vi "Send batch otimizado.vi"() -> ()   [LabVIEW 2018]
panel:
  out "delays":u32[](array[numeric])
  out "responses":string[](array[string])
  in  "instructions":string[](array[string])
  out "error out":errorcluster
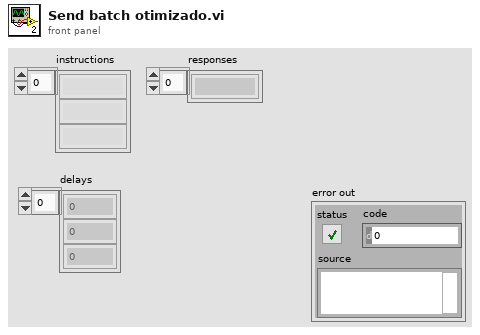
[diagram p1: front panel]
types:
  T1 = enum16{"Standard", "Buffered", "CRLF", "Immediate"}
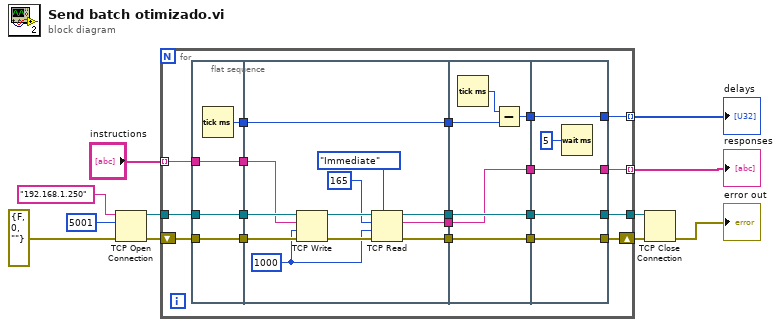
[diagram p0: block diagram]
diagram:
  n1 = TCP Open Connection(address="192.168.1.250" ("motor ip"), remote port or service name=u16 5001 ("motor port"), error in (no error)=errorcluster {"status"=FALSE, "code"=0, "source"=""}) -> (connection ID=w5:refnum<k5>, error out=w9:errorcluster)  [unwired: 2 in]
  n2 = for {
    tunnel: "instructions" -> [w28] mode=indexing
    shift-right: [w12] -> w4
    shift-left: w9 -> [w26]
    tunnel: [w17] -> w10 mode=indexing
    tunnel: w5 -> [w24]
    tunnel: [w20] -> w2
    tunnel: [w19] -> w1 mode=indexing
    n3 = flat-sequence {
      tunnel: [w34] -> w30
      tunnel: w28 -> [w33]
      tunnel: [w33] -> w27
      tunnel: w26 -> [w32]
      tunnel: [w32] -> w25
      tunnel: w24 -> [w31]
      tunnel: [w31] -> w23
      tunnel: [w46] -> w29
      tunnel: w30 -> [w46]
      tunnel: w27 -> [w37]
      tunnel: w25 -> [w42]
      tunnel: w23 -> [w39]
      tunnel: [w41] -> w22
      tunnel: [w38] -> w21
      tunnel: [w35] -> w18
      tunnel: w29 -> [w51]
      tunnel: w22 -> [w49]
      tunnel: w21 -> [w48]
      tunnel: w18 -> [w47]
      tunnel: [w50] -> w16
      tunnel: [w49] -> w15
      tunnel: [w48] -> w14
      tunnel: [w47] -> w13
      tunnel: [w54] -> w19
      tunnel: [w55] -> w20
      tunnel: [w56] -> w12
      tunnel: [w57] -> w17
      tunnel: w16 -> [w57]
      tunnel: w15 -> [w56]
      tunnel: w14 -> [w55]
      tunnel: w13 -> [w54]
      frame #0 {
        n4 = Tick Count (ms)() -> (millisecond timer value=w34:u32)
      }
      frame #1 {
        w36 = 1000 ("timeout ms (60000)")
        n5 = TCP Write(connection ID=w39, data in=w37, error in (no error)=w42, 9:w36) -> (connection ID out=w45:refnum<k5>, error out=w43:errorcluster)  [unwired: 1 out]
        n6 = TCP Read(connection ID=w45, bytes to read=165, error in (no error)=w43, 7:T1."Immediate" ("mode (standard)"), 9:w36) -> (connection ID out=w38:refnum<k5>, data out=w35:string, error out=w41:errorcluster)
      }
      frame #2 {
        n7 = Tick Count (ms)() -> (millisecond timer value=w52:u32)
        n8 = Subtract(x=w52, y=w51) -> (x-y=w50:u32)
      }
      frame #3 {
        n9 = Wait (ms)(milliseconds to wait=u32 5) -> ()  [unwired: 1 out]
      }
    }
  }
  "responses" <- w1
  "delays" <- w10
  n10 = TCP Close Connection(connection ID=w2, error in (no error)=w4) -> (error out=→"error out":errorcluster)  [unwired: 1 in, 1 out]
